vi "Transfer Global Comms Values.vi"(8 "error in (no error)":errorcluster, 10 "Old Service in":refnum<class "Service Action Base.lvclass">, 11 "Service Action Base in":refnum<class "Service Action Base.lvclass">) -> (0 "error out":errorcluster, 3 "Service Action Base out":refnum<class "Service Action Base.lvclass">)   [LabVIEW 2016, in "Assert API Components.lvlib" / "Assert Service.lvlib" / "Service Action Base.lvclass"]
doc: "Used when changing from one type of service class to another, the global values (such as port count) need to be transferred into the new type of class."
uses:
  Service Action Base.lvclass
  Service Action Base.lvclass/Service Action Base.ctl
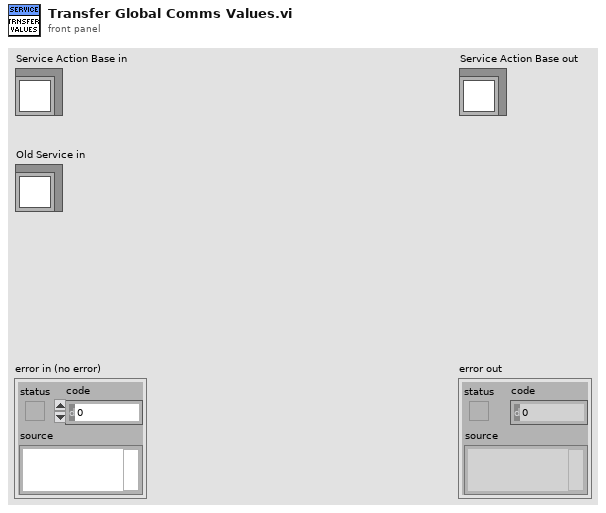
[diagram p1: front panel]
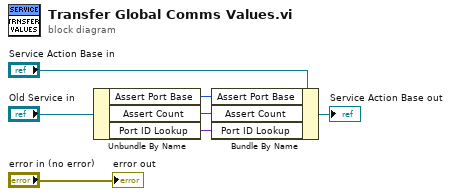
[diagram p0: block diagram]
diagram:
  n1 = Unbundle By Name("Old Service in") -> ("Assert Port Base"=w3:u16, "Assert Count"=w2:u16, "Port ID Lookup"=w1:variant)
  n2 = Bundle By Name(cluster="Service Action Base in", "Assert Port Base"=w3, "Assert Count"=w2, "Port ID Lookup"=w1) -> (→"Service Action Base out":refnum<class "Service Action Base.lvclass">)
  "error out" <- "error in (no error)"
